vi "FTW-Endpoint-ZMQCore-Receive-Multipart.vi"(0 "ØMQ Socket Pointer":u64 format="%016x", 5 "Timeout":i32 format="%dmsec", 11 "error in":errorcluster) -> (4 "ØMQ Socket Pointer out":u64 format="%016x", 6 "Multipart Message":string[](array[string]), 8 "Timed out?":bool, 15 "error out":errorcluster)   [LabVIEW 2012, in "FTW-Actor.lvlib" / "FTW-Endpoint-ZMQ.lvclass"]
uses:
  FTW-Endpoint-ZMQ.lvclass
panel:
  # "Inputs"
  # "Outputs"
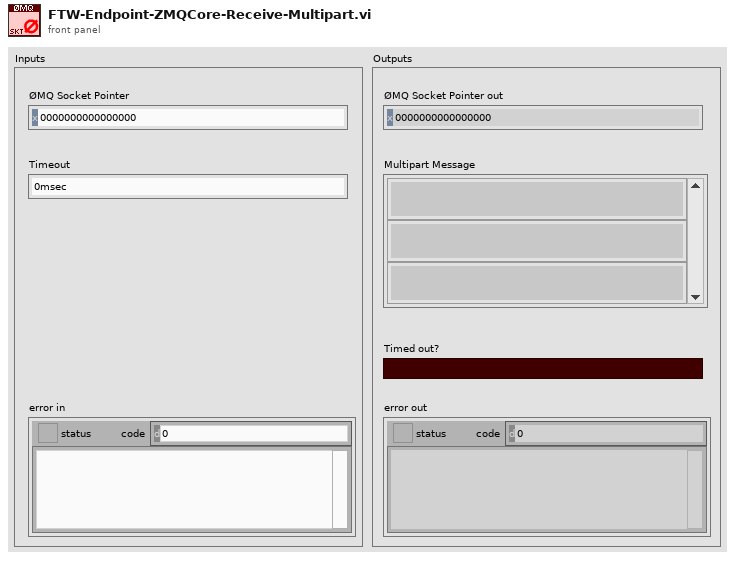
[diagram p1: front panel]
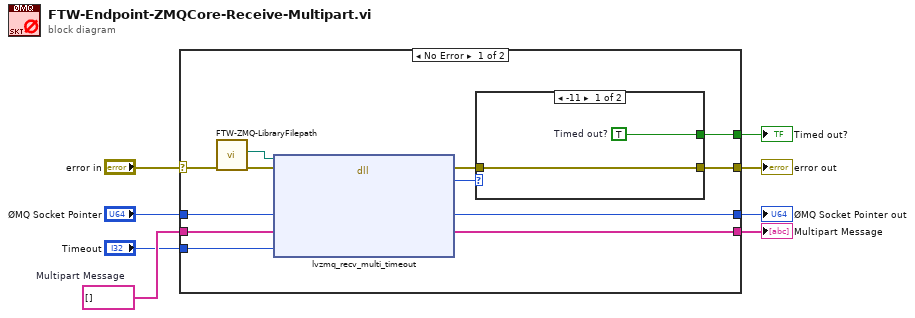
[diagram p0: block diagram]
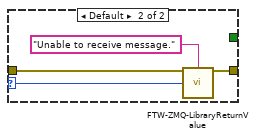
[diagram p2: hidden frame]
diagram:
  w4 = string[] []  # Multipart Message
  n1 = case shown="No Error" "error in" {
    selector: "error in" -> [w11 w28]
    tunnel: "ØMQ Socket Pointer" -> [w14 w29]
    tunnel: [w13 w28] -> w7
    tunnel: [w9 w29] -> w6
    tunnel: w4 -> [w16 w27]
    tunnel: [w15 w27] -> w3
    tunnel: [w12 _] -> w2
    tunnel: "Timeout" -> [w10 _]
    frame No Error {
      n2 = call "FTW-ZMQ-LibraryFilepath.vi"("error in"=w11) -> ("error out"=w18:errorcluster, "FTW-ZMQ Library Filepath"=w17:path)  [unwired: 8 in, 1 out]
      n3 = dll-call lib="?" fn="lvzmq_recv_multi_timeout" ("zmq_labview.dll:lvzmq_socket")(path in=w17, error in=w18, "Socket Pointer"=w14, "Multipart Message"=w16, "Timeout"=w10) -> (error out=w20:errorcluster, "Return Value"=w19:i32, "Socket Pointer"=w9:u64, "Multipart Message"=w15:string[])  [unwired: 4 in, 1 out]
      n4 = case shown="-11" w19 {
        selector: w19 -> [_ w25]
        tunnel: [w22 w23] -> w13
        tunnel: w20 -> [w22 w26]
        tunnel: [w21 _] -> w12
        frame -11 {
          w21 = TRUE  # Timed out?
        }
        frame Default {
          n5 = call "FTW-ZMQ-LibraryReturnValue.vi"("error in"=w26, "Error Message"="Unable to receive message.", "Return Value"=w25) -> ("error out"=w23:errorcluster)  [unwired: 12 in]
        }
      }
    }
    frame Error {
    }
  }
  "error out" <- w7
  "ØMQ Socket Pointer out" <- w6
  "Multipart Message" <- w3
  "Timed out?" <- w2
